vi "apply_password_and_remove_bd.vi"() -> ()   [LabVIEW 2020]
panel:
  in  "Apply Password":bool
  out "error out":errorcluster
  in  "Remove Diagram":bool=TRUE
  in  "Password":string="Iam$oliton"
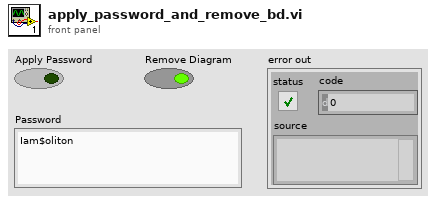
[diagram p1: front panel]
types:
  T1 = enum32{"invalid lock state", "Not Locked", "Locked (No Password)", "Password-protected"}
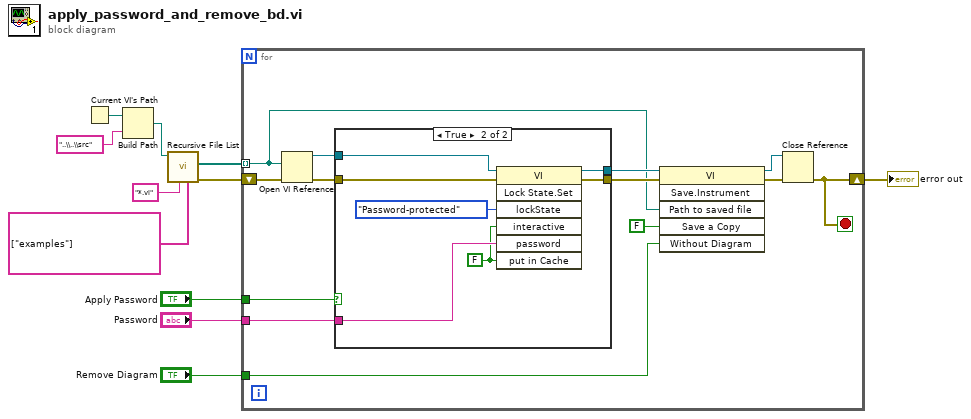
[diagram p0: block diagram]
diagram:
  n1 = Current VI's Path() -> (path=w11:path)
  n2 = Build Path(base path=w11, name or relative path="..\\..\\src") -> (appended path=w9:path)
  n3 = call <vilib>:"Recursive File List.vi"("Folders to Exclude"=string[] ["examples"], "pattern"="*.vi", "Folder Path"=w9) -> ("error out"=w1:errorcluster, "All Files in Dir"=w6:path[])  [unwired: 4 in, 3 out]
  n4 = for {
    tunnel: w6 -> [w18] mode=indexing
    tunnel: "Password" -> [w21]
    tunnel: "Remove Diagram" -> [w16]
    tunnel: "Apply Password" -> [w13]
    shift-right: [w12] -> w3
    shift-left: w1 -> [w24]
    stop <- w12 stop-if-true
    n5 = Open VI Reference(vi path=w18, error in (no error)=w24) -> (vi reference=w22:refnum<vi>, error out=w23:errorcluster)  [unwired: 4 in]
    n6 = case shown="True" w13 {
      tunnel: w23 -> [w26 w33]
      tunnel: w22 -> [w25 w32]
      tunnel: w21 -> [_ w30]
      tunnel: [w26 w28] -> w20
      tunnel: [w25 w27] -> w19
      frame False {
      }
      frame True {
        w29 = FALSE ("Put in Cache")
        n7 = invoke class="VI" method="Lock State.Set"(reference=w32, error in=w33, "lockState"=T1."Password-protected" ("Lock State"), "interactive"=w29, "password"=w30, "put in Cache"=w29) -> (reference out=w27:refnum<vi>, error out=w28:errorcluster)  [unwired: 1 in, 5 out]
      }
    }
    n8 = invoke class="VI" method="Save.Instrument"(reference=w19, error in=w20, "Path to saved file"=w18, "Save a Copy"=FALSE, "Without Diagram"=w16) -> (reference out=w14:refnum<vi>, error out=w15:errorcluster)  [unwired: 1 in, 4 out]
    n9 = Close Reference(reference=w14, error in (no error)=w15) -> (error out=w12:errorcluster)
  }
  "error out" <- w3
